vi "NI_DMM_MODIFIED.vi"(0 "Waveform Points":i32=500 caption="Samples", 1 "Rate":dbl=1800000.0 caption="Rate (Samples/Sec)" format="%.2f", 5 "error in":errorcluster, 7 "close (T)":bool=TRUE caption="close in") -> (14 "Waveform Data":waveform(dbl), 16 "current time":timestamp, 19 "error out":errorcluster)   [LabVIEW 2013]
doc: "Configures and acquires a signal using NI-DMM with National Instruments digital multimeters (DMMs) and NI multiplexer switch modules. NI 4050 and NI 4060 DMMs are not supported by this VI.\n\n<B>Block Diagram Inputs</B>\n\n<B>close (T)</B> - Determines whether the device handle remains open when the VI finishes execution. Use this parameter for loop optimization by setting it to FALSE on all iterations other than the last iteration. When set to TRUE, all references are closed and device is reinitialized in each iteration. <B>close</B> is TRUE by default in Express VI configured for finite acquistion, and FALSE for continuous.\n\n\nNote: This input is not intended to be used to share the data handles between Express VIs. If you have a loop containing multiple Express VIs that use the same device, you must wire in TRUE for this input.\n\n<B>error in</B> - Describes error conditions that occurs before this Express VI runs.\n\n<B>Block Diagram Outputs</B>\n\n<B>signal out</B> - Contains the measured value returned from the DMM.\n\n<B>signal out of range?</B> - Returns whether the measurement value is a valid measurement or a value indicating an over-range under-range condition.\n\n<B>error out</B> - Contains error information. If <B>error in</B> indicates that an error occurred before this Express VI ran, <B>error out</B> contains the same error information. Otherwise, <B>error out</B> describes the error status that this Express VI produces."
uses:
  <instrlib>/niDMM/nidmm.llb/niDMM Waveform Function.ctl
  <instrlib>/niDMM/nidmm.llb/niDMM Function.ctl
  <instrlib>/niDMM/nidmm.llb/niDMM Powerline Frequency.ctl
  <instrlib>/niDMM/nidmm.llb/niDMM Control Actions.ctl
  <instrlib>/niDMM/nidmm.llb/niDMM Read Waveform (waveform data).vi
  <instrlib>/niDMM/nidmm.llb/niDMM Configure Measurement Digits.vi
panel:
  in  "Range":dbl=10.0 format="%.2f"
  out "Actual Number Points Read":i32 caption="Actual Number"
  in  "resource name":refnum<k15>="PXI1Slot4"
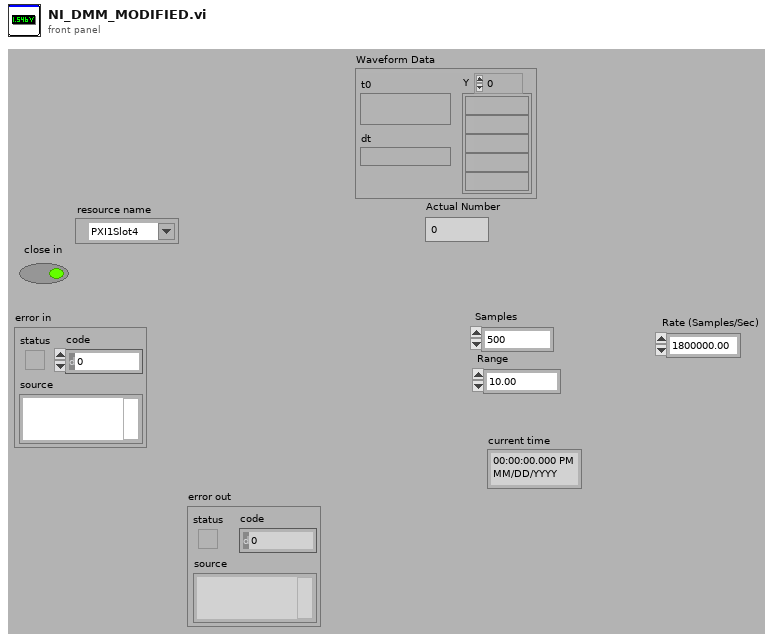
[diagram p1: front panel]
types:
  T1 = typedef "niDMM Waveform Function.ctl" = i32
  T2 = typedef "niDMM Powerline Frequency.ctl" = enum16{"60 Hz", "50 Hz"}
  T3 = typedef "niDMM Function.ctl" = enum16{"DC Volts", "AC Volts", "DC Current", "AC Current", "2-wire Resistance", "4-wire Resistance", "Diode", "Frequency", "Period", "AC Volts DC Coupled", "Capacitance", "Inductance", "Temperature"}
  T4 = typedef "niDMM Control Actions.ctl" = i32
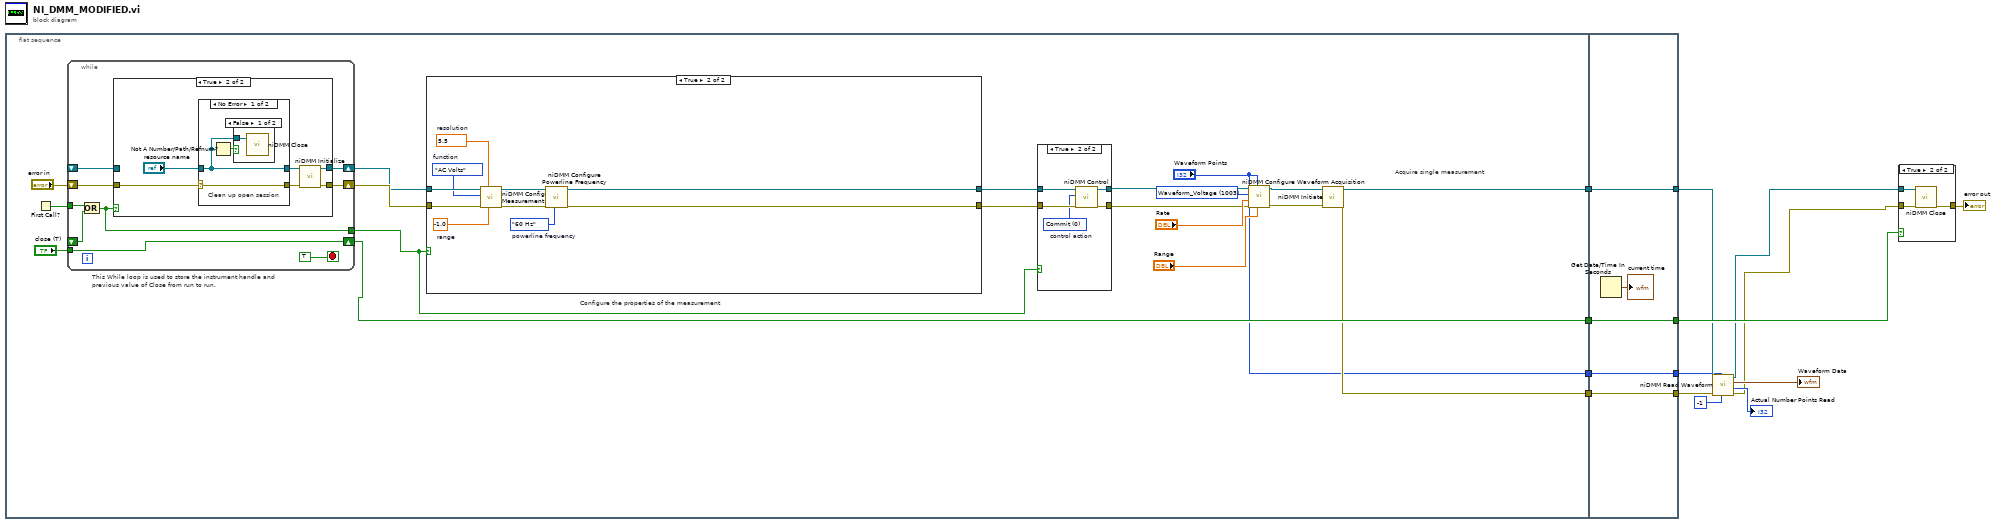
[diagram p0: block diagram]
diagram:
  n1 = flat-sequence {
    tunnel: [w25] -> w6
    tunnel: [w17] -> w5
    tunnel: [w16] -> w4
    tunnel: ["Waveform Points"] -> w3
    tunnel: [w77] -> w7
    tunnel: [w78] -> w9
    tunnel: [w79] -> w10
    tunnel: [w80] -> w13
    tunnel: w6 -> [w80]
    tunnel: w5 -> [w79]
    tunnel: w4 -> [w78]
    tunnel: w3 -> [w77]
    frame #0 {
      w24 = T1 1003 items=["Waveform_Voltage"=1003, "Waveform_Current"=1004] ("Function")
      # "Acquire single measurement"
      # "Configure the properties of the measurement"
      # "This While loop is used to store the instrument handle and previous value of Close from run to run."
      n2 = First Call?() -> (First Call?: T/F=w30:bool)
      n3 = while "Init Loop" {
        shift-right: [w58] -> w29
        shift-left: _ -> [w59]
        shift-right: [w57] -> w31
        shift-left: "error in" -> [w60]
        shift-right: [w55] -> w25
        shift-left: _ -> [w56]
        tunnel: "close (T)" -> [w55]
        tunnel: w30 -> [w54]
        tunnel: [w53] -> w26
        stop <- TRUE stop-if-true
        n4 = Or(x=w54, y=w56) -> (x .or. y?=w53:bool)
        n5 = case "Init Case" shown="True" w53 {
          tunnel: w60 -> [w62 w66]
          tunnel: w59 -> [w63 _]
          tunnel: [w63 w69] -> w58
          tunnel: [w62 w68] -> w57
          frame False {
          }
          frame True {
            n6 = case "Clean up open resource" shown="No Error" w66 {
              selector: w66 -> [w71 w74]
              tunnel: "resource name" -> [w70 w75]
              tunnel: [w70 w75] -> w67
              tunnel: [w71 w74] -> w65
              frame No Error {
                # "Clean up open session"
                n7 = Not A Number/Path/Refnum?(number/path/refnum=w70) -> (NaN/Path/Refnum?=w72:bool)
                n8 = case shown="False" w72 {
                  tunnel: w70 -> [w73 _]
                  frame False {
                    n9 = call <instrlib>:"niDMM Close.vi"("instrument handle"=w73) -> ()  [unwired: 1 in, 10 out]
                  }
                  frame True {
                  }
                }
              }
              frame Error {
              }
            }
            n10 = call <instrlib>:"niDMM Initialize.vi"("error in (no error)"=w65, "Instrument Descriptor"=w67) -> ("error out"=w68:errorcluster, "instrument handle out"=w69:refnum<k15>)  [unwired: 2 in, 6 out]
          }
        }
      }
      n11 = case "Config Case" shown="True" w26 {
        tunnel: w29 -> [w42 w48]
        tunnel: w31 -> [w41 w52]
        tunnel: [w41 w50] -> w28
        tunnel: [w42 w51] -> w27
        frame False {
        }
        frame True {
          w46 = 5.5 items=["3 1/2"=3.5, "4 1/2"=4.5, "5 1/2"=5.5, "6 1/2"=6.5, "7 1/2"=7.5]  # resolution
          w43 = niDMM_Powerline_Frequency."60 Hz"  # powerline frequency
          w45 = -1.0  # range
          w47 = niDMM_Function."AC Volts"  # function
          n12 = call-poly <instrlib>:"niDMM Config Measurement.vi"("Range"=w45, "Resolution in Digits"=w46, "error in (no error)"=w52, "Function"=w47, "instrument handle"=w48) -> ("error out"=w44:errorcluster, "instrument handle out"=w49:refnum<k15>)  [unwired: 5 in]
          n13 = call <instrlib>:"niDMM Configure Powerline Frequency.vi"("Powerline Frequency"=w43, "error in (no error)"=w44, "instrument handle"=w49) -> ("error out"=w50:errorcluster, "instrument handle out"=w51:refnum<k15>)  [unwired: 7 in]
        }
      }
      n14 = case shown="True" w26 {
        tunnel: w28 -> [w34 w40]
        tunnel: w27 -> [w35 w39]
        tunnel: [w35 w38] -> w20
        tunnel: [w34 w37] -> w19
        frame False {
        }
        frame True {
          w36 = T4 0 items=["Commit"]  # control action
          n15 = call <instrlib>:"niDMM Control.vi"("error in (no error)"=w40, "Control Action"=w36, "instrument handle"=w39) -> ("error out"=w37:errorcluster, "instrument handle out"=w38:refnum<k15>)  [unwired: 7 in]
        }
      }
      n16 = call <instrlib>:"niDMM Configure Waveform Acquisition.vi"("Range"="Range", "Waveform Points"="Waveform Points", "error in (no error)"=w19, "Rate"="Rate", "Function"=w24, "instrument handle"=w20) -> ("error out"=w18:errorcluster, "instrument handle out"=w21:refnum<k15>)  [unwired: 4 in]
      n17 = call <instrlib>:"niDMM Initiate.vi"("error in (no error)"=w18, "instrument handle"=w21) -> ("error out"=w16:errorcluster, "instrument handle out"=w17:refnum<k15>)  [unwired: 8 in]
    }
    frame #1 {
      n18 = Get Date/Time In Seconds() -> (seconds since 1Jan1904=→"current time":timestamp)
    }
  }
  n19 = call-poly <instrlib>:"niDMM Read Waveform.vi"("Maximum Time (msec)"=-1, "Number To Read"=w7, "error in (no error)"=w9, "instrument handle"=w10) -> ("error out"=w1:errorcluster, "Actual Number"=→"Actual Number Points Read":i32, "Waveform Data"=→"Waveform Data":waveform(dbl), "instrument handle out"=w2:refnum<k15>)  [unwired: 4 in]
  n20 = case shown="True" w13 {
    tunnel: w1 -> [w81 w84]
    tunnel: [w81 w83] -> w14
    tunnel: w2 -> [_ w82]
    frame False {
    }
    frame True {
      n21 = call <instrlib>:"niDMM Close.vi"("error in (no error)"=w84, "instrument handle"=w82) -> ("error out"=w83:errorcluster)  [unwired: 9 in]
    }
  }
  "error out" <- w14
